vi "Connect OPCUA Server Auto.vi"(4 "timeout (5000 ms)":u32=5000, 7 "username/password":cluster{"username":string, "password":string}, 8 "Error In":errorcluster, 9 "client cert path(empty path)":path, 10 "Server IP":string, 11 "XML config File Path":path=path "D:/work/Project support in lanzhou/OPCUA XML/xml/server config.xml") -> (0 "Error Out":errorcluster, 1 "OPC UA data change event":refnum<user-event>, 2 "server endpoint URL":string, 3 "OPC UA client refnum":refnum<k21>, 5 "trusted Server certfications":path[](array[path]))   [LabVIEW 2014, in "OPCUA XML(dev).lvlib"]
doc: "This example loads test configuration data from an XML file, and checks to see if it is valid against a specific schema. Select whether you want to load the valid or invalid file and run the VI to see the results."
uses:
  OPCUA XML(dev).lvlib
  <vilib>/OPCUA/NI OPC UA Client.lvlib
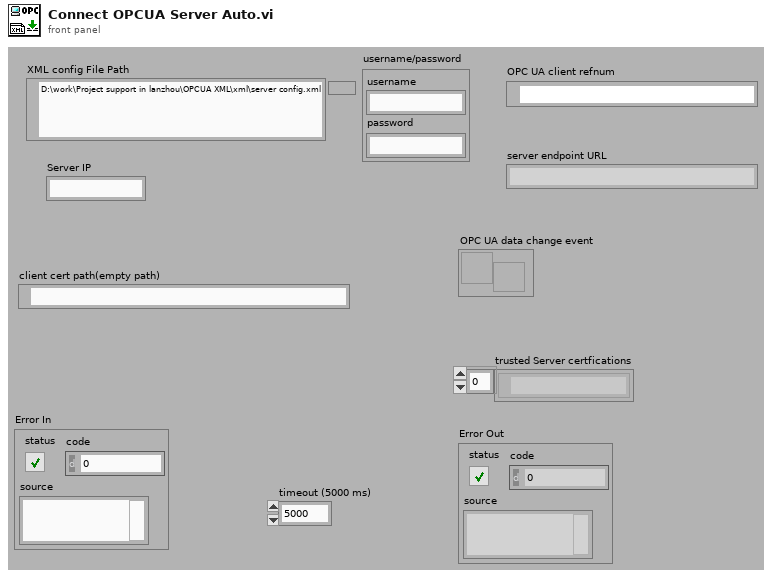
[diagram p1: front panel]
types:
  T1 = typedef "OPCUA XML(dev).lvlib/DEF-Server Config Data.ctl" = cluster{"name data":string, "port data":string, "policy data":string, "serverCertification data":string, "trustedClientCertifications data":string, "structure data":string}
  T2 = cluster{"message mode":enum16{"None", "Sign", "Sign and Encrypt"}, "security":enum16{"Basic256", "Basic128Rsa15"}}
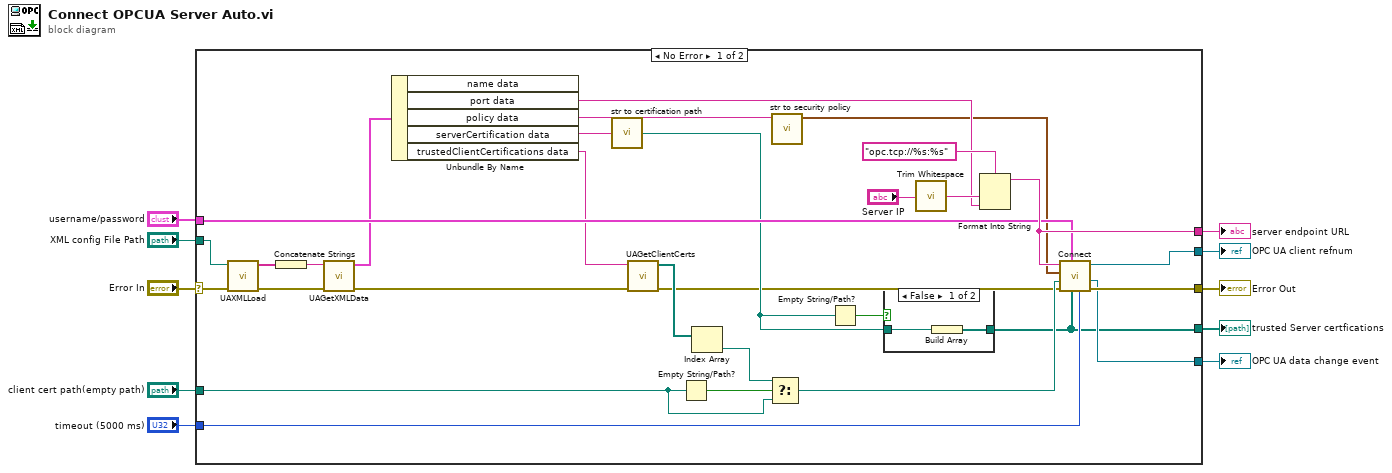
[diagram p0: block diagram]
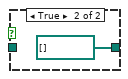
[diagram p2: hidden frame]
diagram:
  n1 = case shown="No Error" "Error In" {
    selector: "Error In" -> [w37 w44]
    tunnel: [w39 w44] -> w3
    tunnel: "XML config File Path" -> [w36 _]
    tunnel: [w40 _] -> w4
    tunnel: [w32 _] -> w5
    tunnel: [w25 _] -> w2
    tunnel: [w38 _] -> w1
    tunnel: "client cert path(empty path)" -> [w30 _]
    tunnel: "username/password" -> [w29 _]
    tunnel: "timeout (5000 ms)" -> [w28 _]
    frame No Error {
      n2 = call "UAXMLLoad.vi"("error in (no error)"=w37, "XML File Path"=w36) -> ("error out"=w23:errorcluster, "xml Data"=w24:string[])  [unwired: 8 in]
      n3 = Concatenate Strings(w24) -> (w22:string)
      n4 = call "UAGetXMLData.vi"("error in (no error)"=w23, "String"=w22) -> ("error out"=w12:errorcluster, "Server config info"=w21:T1)  [unwired: 8 in]
      n5 = Unbundle By Name(w21) -> ("port data"=w20:string, "policy data"=w19:string, "serverCertification data"=w17:string, "trustedClientCertifications data"=w15:string)  [unwired: 1 out]
      n6 = call "str to certification path.vi"("node text"=w17) -> ("File Path Control"=w16:path)  [unwired: 4 in]
      n7 = call "UAGetClientCerts.vi"("error in (no error)"=w12, "trustedClientCertifications data"=w15) -> ("error out"=w11:errorcluster, "Array"=w14:path[])  [unwired: 8 in]
      n8 = Empty String/Path?(string/path=w30) -> (empty?=w31:bool)
      n9 = Index Array(array=w14) -> (element=w13:path)  [unwired: 1 in]
      n10 = Select(t=w13, s=w31, f=w30) -> (s? t:f=w27:path)
      n11 = call "str to security policy.vi"("trimmed string"=w19) -> ("security policy"=w18:T2)  [unwired: 10 in]
      n12 = Empty String/Path?(string/path=w16) -> (empty?=w26:bool)
      n13 = case shown="False" w26 {
        tunnel: w16 -> [w42 _]
        tunnel: [w41 path[] []] -> w25
        frame False {
          n14 = Build Array(w42) -> (w41:path[])
        }
        frame True {
        }
      }
      n15 = call <vilib>:"Trim Whitespace.vi"("string"="Server IP") -> ("trimmed string"=w34:string)  [unwired: 1 in]
      n16 = Format Into String(format string="opc.tcp://%s:%s", w34, w20) -> (resulting string=w32:string)  [unwired: 2 in, 1 out]
      n17 = call <vilib>:"Connect.vi"("timeout (5000 ms)"=w28, "trusted server certificates"=w25, "username/password"=w29, "error in (no error)"=w11, "client certificate file"=w27, "security policy"=w18, "server endpoint URL"=w32) -> ("error out"=w39:errorcluster, "OPC UA data change event"=w38:refnum<user-event>, "OPC UA client refnum out"=w40:refnum<k21>)  [unwired: 2 in]
    }
    frame Error {
    }
  }
  "Error Out" <- w3
  "server endpoint URL" <- w5
  "trusted Server certfications" <- w2
  "OPC UA client refnum" <- w4
  "OPC UA data change event" <- w1
